vi "generate adjusted img for optimization (SubVI).vi"(10 "data":variant, 11 "X":dbl[](array[numeric])) -> (0 "error out":errorcluster, 2 "Array":dbl[][](array[numeric]), 3 "GT":dbl[][](array[numeric]))   [LabVIEW 2024]
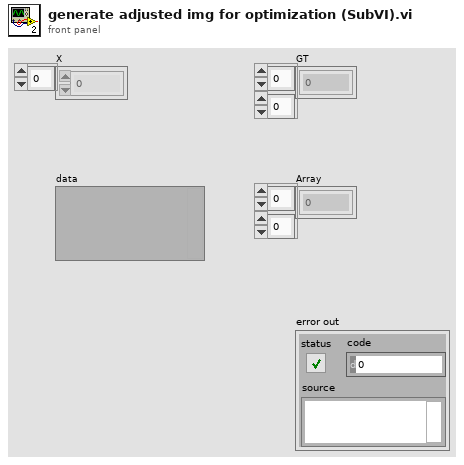
[diagram p1: front panel]
types:
  T1 = cluster{"GT":dbl[][], "frame input":u16[][], "cut pos init":dbl, "Nx":dbl, "r init":dbl}
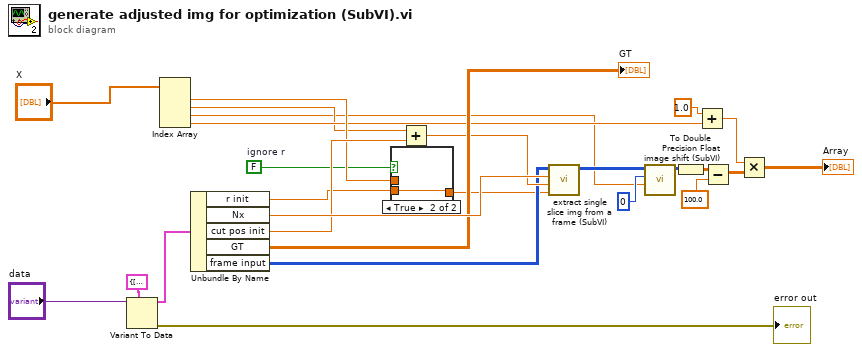
[diagram p0: block diagram]
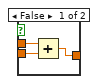
[diagram p2: hidden frame]
diagram:
  w2 = FALSE  # ignore r
  n1 = Variant To Data(type=T1 {"GT"=[], "frame input"=[], "cut pos init"=0.0, "Nx"=0.0, "r init"=0.0}, Variant="data") -> (data=w18:T1, error out=→"error out":errorcluster)  [unwired: 1 in]
  n2 = Index Array(array="X") -> (element #1=w21:dbl, element #2=w5:dbl, element #3=w4:dbl, element #4=w7:dbl)  [unwired: 4 in]
  n3 = Unbundle By Name(w18) -> ("r init"=w3:dbl, "Nx"=w25:dbl, "cut pos init"=w24:dbl, "GT"=→"GT":dbl[][], "frame input"=w19:u16[][])
  n4 = case shown="True" w2 {
    tunnel: w21 -> [w29 _]
    tunnel: w3 -> [w28 w30]
    tunnel: [w27 w30] -> w1
    frame False {
      n5 = Add(x=w29, y=w28) -> (x+y=w27:dbl)
    }
    frame True {
    }
  }
  n6 = Add(x=w5, y=w24) -> (x+y=w22:dbl)
  n7 = call "extract single slice img from a frame (SubVI).vi"("AOD scan speed ratio"=w1, "init pos"=w22, "Nx"=w25, "image in"=w19) -> ("Array"=w14:u16[][])  [unwired: 7 in]
  n8 = call "image shift (SubVI).vi"("v shift"=w4, "h shift"=0, "Array in"=w14) -> ("Array out"=w13:u16[][])  [unwired: 8 in]
  n9 = To Double Precision Float(number=w13) -> (double precision float=w12:dbl[][])
  n10 = Add(x=1.0 ("element"), y=w7) -> (x+y=w8:dbl)
  n11 = Subtract(x=w12, y=100.0) -> (x-y=w15:dbl[][])
  n12 = Multiply(x=w8, y=w15) -> (x*y=→"Array":dbl[][])
